vi "Stoerungs-Queue in Tabelle Stoermeldungen.vi"(6 "Abschalten aus Datei":bool[](array[boolean]), 9 "Störmeldetexte aus Datei":string[](array[string]), 10 "Quittieren aus Datei":bool[](array[boolean]), 11 "Queue-Inhalt\n(FGV Störmeldungen)":T1[](array[typedef])) -> (1 "Störungsnummern":i32[](array[numeric]), 3 "Tabelle Störmeldungen":string[][](array[string]))   [LabVIEW 2020, in "Stoerungen.lvlib"]
uses:
  Stoerungen.lvlib
  Stoermeldung.ctl
  Sprachverwaltung/FGV Aktion Tabelle zerlegen.ctl
  Sprachverwaltung/Sprachverwaltung.lvlib
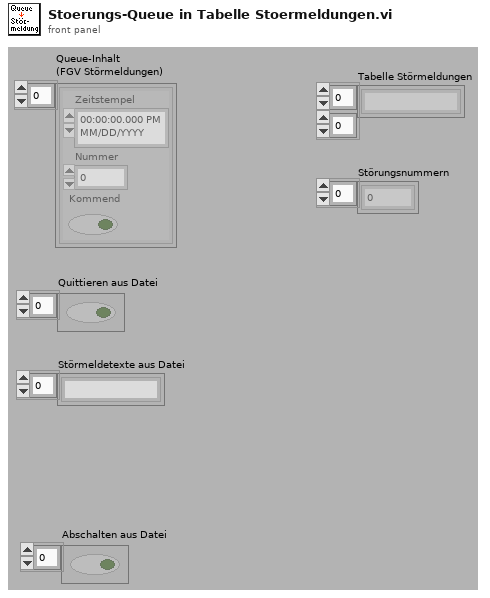
[diagram p1: front panel]
types:
  T1 = typedef "Stoerungen.lvlib/Stoermeldung.ctl" = cluster{"Zeitstempel":timestamp, "Nummer":i32, "Kommend":bool}
  T2 = typedef "Sprachverwaltung.lvlib/FGV Aktion Tabelle zerlegen.ctl" = enum16{"laden", "vereinzeln", "speichern"}
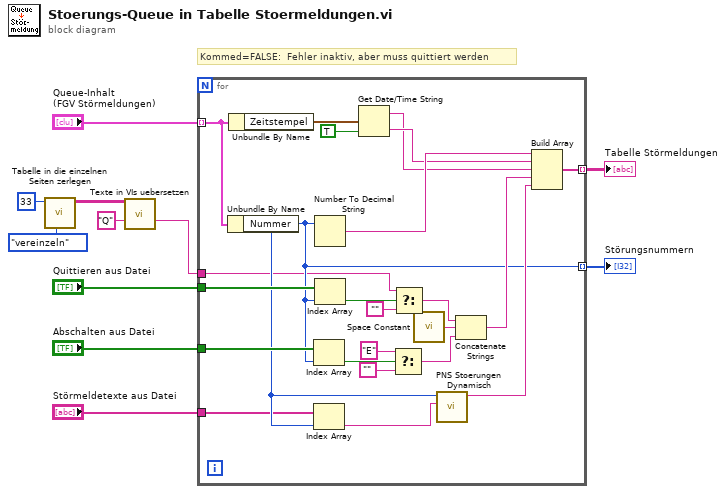
[diagram p0: block diagram]
diagram:
  # "Kommed=FALSE:  Fehler inaktiv, aber muss quittiert werden"
  n1 = call "Tabelle in die einzelnen Seiten zerlegen.vi"("Aktion"=FGV_Aktion_Tabelle_zerlegen."vereinzeln", "Index (Seite)"=33) -> ("Sprachliste"=w3:string[][])  [unwired: 7 in, 2 out]
  n2 = call "Texte in VIs uebersetzen.vi"("Sprachliste"=w3, "String zum Übersetzen"="Q") -> ("String zum Übersetzen"=w1:string)  [unwired: 9 in, 4 out]
  n3 = for {
    tunnel: "Störmeldetexte aus Datei" -> [w13]
    tunnel: "Quittieren aus Datei" -> [w29]
    tunnel: "Queue-Inhalt\n(FGV Störmeldungen)" -> [w27] mode=indexing
    tunnel: [w26] -> w10 mode=indexing
    tunnel: [w15] -> w8 mode=indexing
    tunnel: "Abschalten aus Datei" -> [w24]
    tunnel: w1 -> [w12]
    n4 = Unbundle By Name(w27) -> ("Nummer"=w15:i32)
    n5 = Unbundle By Name(w27) -> ("Zeitstempel"=w34:timestamp)
    n6 = Index Array(array=w24, index=w15) -> (element=w21:bool)
    n7 = Index Array(array=w13, index=w15) -> (element=w14:string)
    n8 = Number To Decimal String(number=w15) -> (decimal integer string=w32:string)  [unwired: 1 out]
    n9 = Index Array(array=w29, index=w15) -> (element=w28:bool)
    n10 = Get Date/Time String(seconds (now)=w34, want seconds? (F)=TRUE ("Angabe von Sekunden? (F)")) -> (date string=w30:string, time string=w31:string)  [unwired: 1 out]
    n11 = Select(t="E" ("f"), s=w21, f="") -> (s? t:f=w19:string)
    n12 = Select(t=w12, s=w28, f="") -> (s? t:f=w20:string)
    n13 = call <vilib>:"Space Constant.vi"() -> ("String"=w18:string)
    n14 = call "PNS Stoerungen Dynamisch.vi"("Störmeldetexte"=w14, "Nummer"=w15) -> ("String"=w16:string)  [unwired: 9 in]
    n15 = Concatenate Strings(w20, w18, w19) -> (w17:string)
    n16 = Build Array(w32, w31, w30, w17, w16) -> (w26:string[])
  }
  "Tabelle Störmeldungen" <- w10
  "Störungsnummern" <- w8
